vi "Update Zones Booleans.vi"(8 "error in (no error)":errorcluster, 11 "PL Model Data":T1={"Position"=0.0, "Settings"={"Length [m]"=20.0, "Dose Zone Start"=8.0, "Dose Zone  End"=12.0, "Barrel Volume [l]"=100.0, "Dosing level [l]"=90.0}, "Pump State"=FALSE, "Fluid Flow"=0.0, "Inpute Zone"=FALSE, "Dosing Zone"=FALSE, "Output Zone"=FALSE, "UI Refs"={"DOSING"=refnum, "INPUT"=refnum, "OUTPUT"=refnum, "Pump"=refnum, "Fluid Level [l]"=refnum, "Flow [l/s]"=refnum, "Production line"=refnum, "SPILL"=refnum, "LOW LEVEL"=refnum, "Barrel Number"=refnum}, "Fluid Level"=0.0, "Barrel Number"=0, "Spill Alarm"=FALSE, "Level Alarm"=FALSE, "millisecond timer value"=0}) -> (0 "error out":errorcluster, 2 "Zone change?":bool, 3 "PL Model Data 2":T1={"Position"=0.0, "Settings"={"Length [m]"=20.0, "Dose Zone Start"=8.0, "Dose Zone  End"=12.0, "Barrel Volume [l]"=100.0, "Dosing level [l]"=90.0}, "Pump State"=FALSE, "Fluid Flow"=0.0, "Inpute Zone"=FALSE, "Dosing Zone"=FALSE, "Output Zone"=FALSE, "UI Refs"={"DOSING"=refnum, "INPUT"=refnum, "OUTPUT"=refnum, "Pump"=refnum, "Fluid Level [l]"=refnum, "Flow [l/s]"=refnum, "Production line"=refnum, "SPILL"=refnum, "LOW LEVEL"=refnum, "Barrel Number"=refnum}, "Fluid Level"=0.0, "Barrel Number"=0, "Spill Alarm"=FALSE, "Level Alarm"=FALSE, "millisecond timer value"=0})   [LabVIEW 2015, in "PL Model.lvlib"]
uses:
  PL Model.lvlib
  TypeDefs/PL Settings.ctl
  TypeDefs/PL UI Refs.ctl
  TypeDefs/PL Model Data.ctl
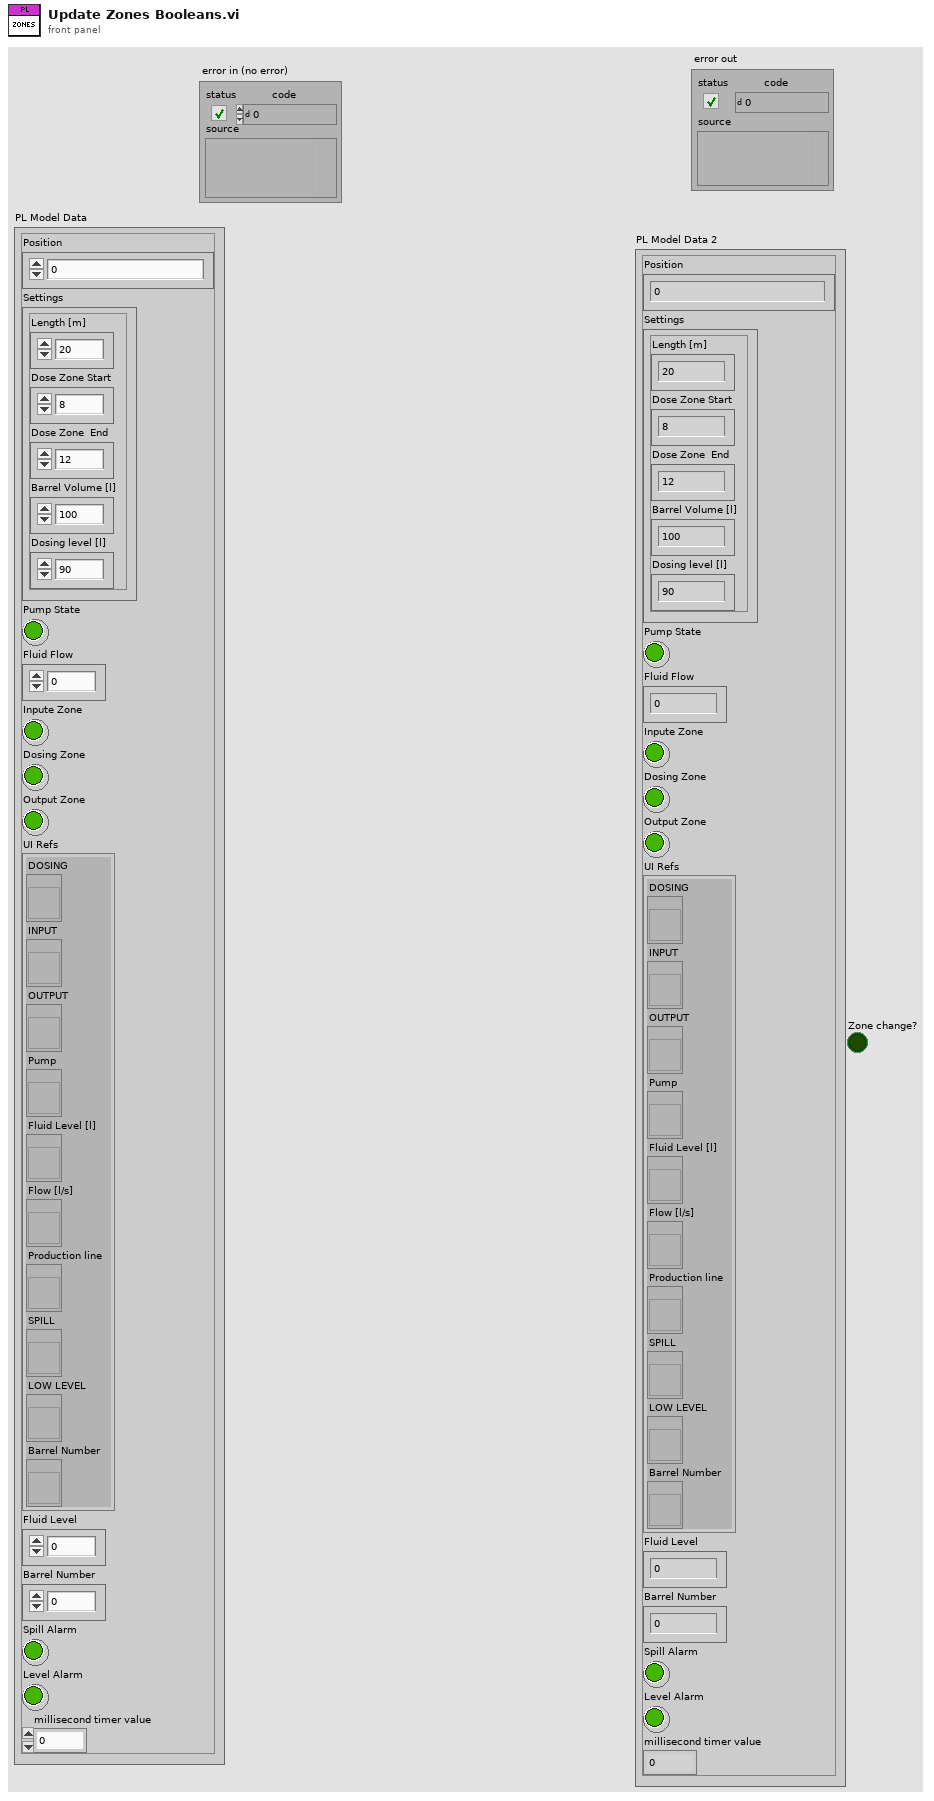
[diagram p1: front panel]
types:
  T1 = typedef "PL Model.lvlib/PL Model Data.ctl" = cluster{"Position":dbl, "Settings":T2, "Pump State":bool, "Fluid Flow":dbl, "Inpute Zone":bool, "Dosing Zone":bool, "Output Zone":bool, "UI Refs":T3, "Fluid Level":dbl, "Barrel Number":i32, "Spill Alarm":bool, "Level Alarm":bool, "millisecond timer value":u32}
  T2 = typedef "PL Model.lvlib/PL Settings.ctl" = cluster{"Length [m]":dbl, "Dose Zone Start":dbl, "Dose Zone  End":dbl, "Barrel Volume [l]":dbl, "Dosing level [l]":dbl}
  T3 = typedef "PL Model.lvlib/PL UI Refs.ctl" = cluster{"DOSING":refnum<vi>, "INPUT":refnum<vi>, "OUTPUT":refnum<vi>, "Pump":refnum<vi>, "Fluid Level [l]":refnum<vi>, "Flow [l/s]":refnum<vi>, "Production line":refnum<vi>, "SPILL":refnum<vi>, "LOW LEVEL":refnum<vi>, "Barrel Number":refnum<vi>}
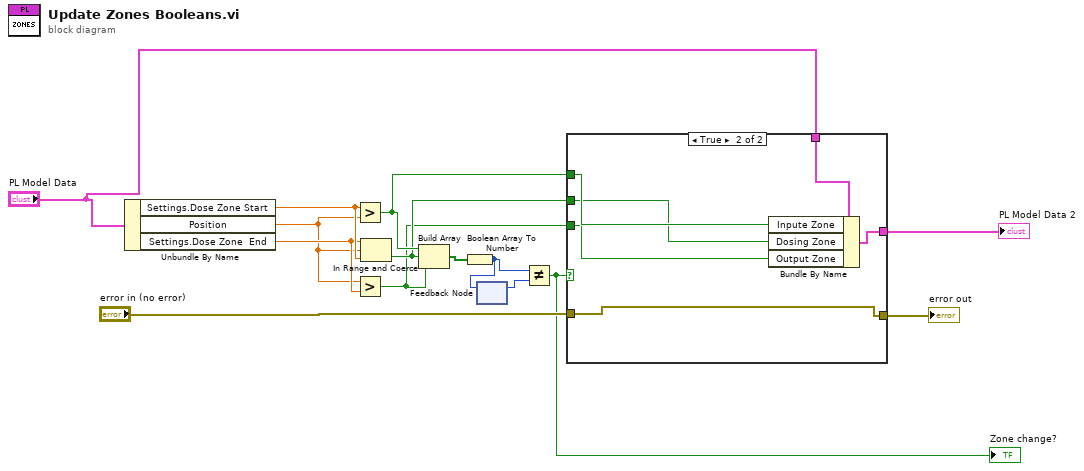
[diagram p0: block diagram]
diagram:
  n1 = Unbundle By Name("PL Model Data") -> ("Settings.Dose Zone Start"=w14:dbl, "Position"=w12:dbl, "Settings.Dose Zone  End"=w13:dbl)
  n2 = Greater?(x=w14, y=w12) -> (0:w4:bool)
  n3 = Greater?(x=w12, y=w13) -> (0:w2:bool)
  n4 = In Range and Coerce(upper limit=w13, x=w12, lower limit=w14) -> (In Range?=w3:bool)  [unwired: 1 out]
  n5 = Build Array(w4, w3, w2) -> (w5:bool[])
  n6 = Boolean Array To Number(Boolean array=w5) -> (number=w9:u32)
  n7 = feedback-in #1(w9) -> ()
  n8 = feedback #1() -> (w8:u32)  [unwired: 1 in]
  n9 = Not Equal?(x=w9, y=w8) -> (x != y?=w7:bool)
  "Zone change?" <- w7
  n10 = case shown="True" w7 {
    tunnel: "error in (no error)" -> [w16 w17]
    tunnel: [w16 w17] -> w10
    tunnel: "PL Model Data" -> [w15 w22]
    tunnel: w4 -> [_ w21]
    tunnel: w3 -> [_ w20]
    tunnel: w2 -> [_ w19]
    tunnel: [w15 w18] -> w1
    frame False {
    }
    frame True {
      n11 = Bundle By Name(cluster=w22, "Inpute Zone"=w21, "Dosing Zone"=w20, "Output Zone"=w19) -> (w18:T1)
    }
  }
  "PL Model Data 2" <- w1
  "error out" <- w10
